vi "merFISH_scan_single_step.vi"(3 "iteration":i32, 4 "queue DAQ":refnum<queue>, 5 "error in":errorcluster, 6 "Z position":dbl, 7 "# steps":i32, 8 "queue piezo":refnum<queue>) -> (0 "error out":errorcluster)   [LabVIEW 2015]
uses:
  CONTROLS/Q_MCL_piezo_element.ctl
  CONTROLS/Q_DAQ_element.ctl
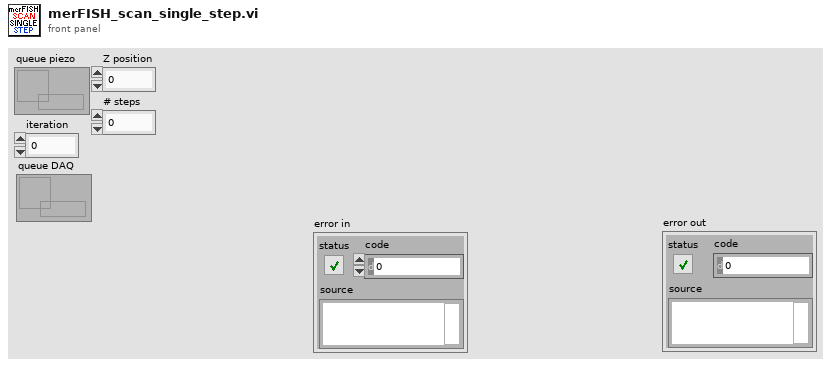
[diagram p1: front panel]
types:
  T1 = typedef "Q_DAQ_element.ctl" = cluster{"variant":variant, "Instruction":enum16{"DAQ_idle", "DAQ_initialize", "DAQ_error", "DAQ_security_stop", "DAQ_init_single_scan", "DAQ_single_scan", "DAQ_init_merFISH", "DAQ_scan_merFISH", "DAQ_photobleaching_merFISH", "DAQ_close_merFISH", "DAQ_stop"}}
  T2 = cluster{"iteration":i32, "# steps":i32, "Z position":dbl}
  T3 = typedef "Q_MCL_piezo_element.ctl" = cluster{"variant":variant, "Instruction":enum16{"Piezo_idle", "Piezo_initialize", "Piezo_error", "Piezo_security_stop", "Piezo_read_z", "Piezo_move_z", "Piezo_keyboard_move", "Piezo_close_autofocus_calibration_ramp", "Piezo_change_init_state", "Piezo_init_autofocus", "Piezo_init_autofocus_merFISH_TL", "Piezo_autofocus", "Piezo_autofocus_merFISH_TL", "Piezo_stop_autofocus", "Piezo_stop_autofocus_merFISH_TL", "Piezo_autofocus_lost", "Piezo_resume_autofocus_merFISH_TL", "Piezo_check_z_position_merFISH_TL", "Piezo_init_ramp", "Piezo_move_z_ramp", "Piezo_close_ramp", "Piezo_close_merFISH", "Piezo_stop"}}
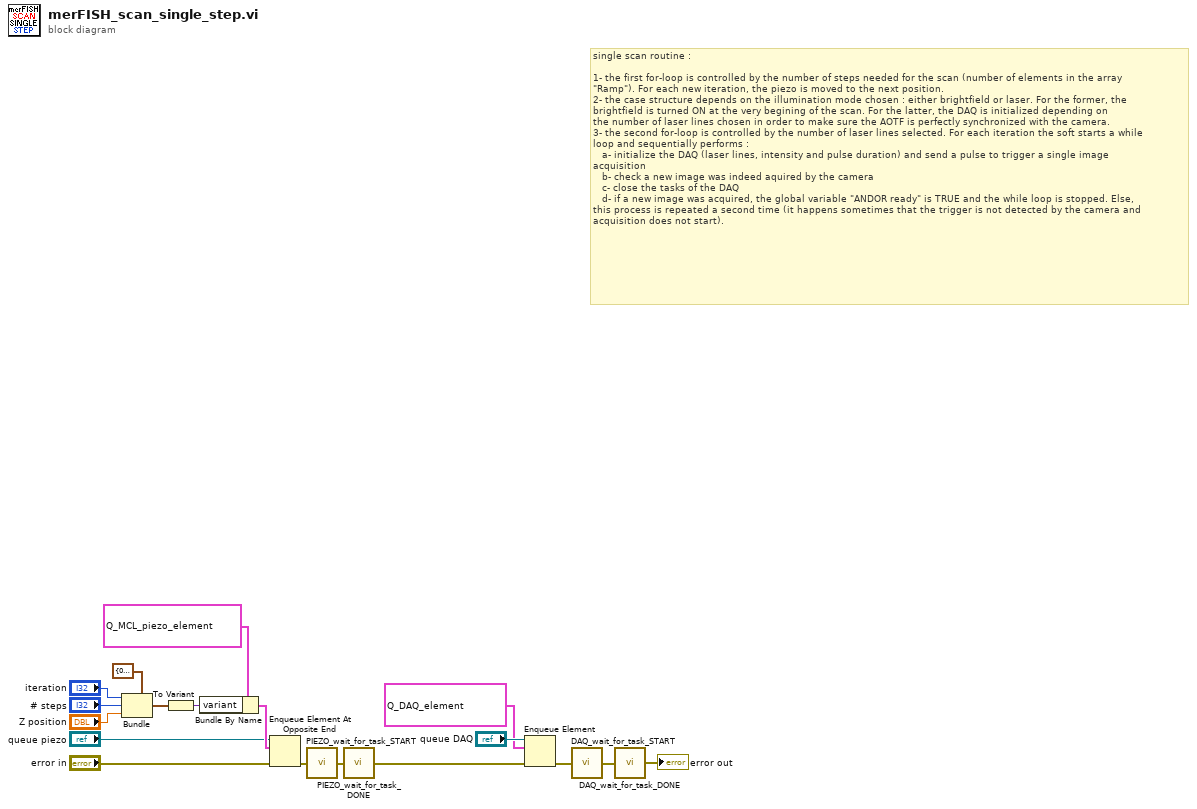
[diagram p0: block diagram]
diagram:
  # "single scan routine :\n\n1- the first for-loop is controlled by the number of steps needed for the scan (number of elements in the array\n\"Ramp\"). For each new iteration, the piezo is moved to the next position.\n2- the case structure depends on the illumination mode chosen : either brightfield or laser. For the former, the\nbrightfield is turned ON at the very begining of the scan. For the latter, the DAQ is initialized depending on\nthe number of laser lines chosen in order to make sure the AOTF is perfectly synchronized with the camera.\n3- the second for-loop is controlled by the number of laser lines selected. For each iteration the soft starts a while\nloop and sequentially performs :\n   a- initialize the DAQ (laser lines, intensity and pulse duration) and send a pulse to trigger a single image\nacquisition\n   b- check a new image was indeed aquired by the camera\n   c- close the tasks of the DAQ\n   d- if a new image was acquired, the global variable \"ANDOR ready\" is TRUE and the while loop is stopped. Else, \nthis process is repeated a second time (it happens sometimes that the trigger is not detected by the camera and\nacquisition does not start)."
  n1 = Bundle(cluster=T2 {"iteration"=0, "# steps"=0, "Z position"=0.0} ("output cluster"), "iteration"="iteration", "# steps"="# steps", "Z position"="Z position") -> (w15:T2)
  n2 = To Variant(anything=w15) -> (Variant=w11:variant)
  n3 = Bundle By Name(cluster=T3 {"variant"=variant, "Instruction"=enum."Piezo_move_z_ramp"} ("Q_MCL_Piezo"), "variant"=w11) -> (w12:T3)
  n4 = Enqueue Element At Opposite End(queue="queue piezo", element=w12, error in (no error)="error in") -> (error out=w13:errorcluster)  [unwired: 1 in, 2 out]
  n5 = call "PIEZO_wait_for_task_START.vi"("error in"=w13) -> ("error out"=w14:errorcluster)
  n6 = call "PIEZO_wait_for_task_DONE.vi"("error in"=w14) -> ("error out"=w16:errorcluster)
  n7 = Enqueue Element(queue="queue DAQ", element=T1 {"variant"=variant, "Instruction"=enum."DAQ_single_scan"}, error in (no error)=w16) -> (error out=w17:errorcluster)  [unwired: 1 in, 2 out]
  n8 = call "DAQ_wait_for_task_START.vi"("error in"=w17) -> ("error out"=w18:errorcluster)
  n9 = call "DAQ_wait_for_task_DONE.vi"("error in"=w18) -> ("error out"=→"error out":errorcluster)
